vi "WPI_AnalogChannelVoltageToValue.vi"(6 "Relative":bool, 8 "error in (no error)":errorcluster, 9 "Averaged":bool, 10 "Voltage":dbl, 11 "AIDeviceRef":T1={"DevStatus"={"status"=FALSE, "code"=0, "source"=""}, "Analog Channel"=enum."AI 1"}) -> (0 "error out":errorcluster, 2 "Value":i32, 3 "AIDeviceRef":T1={"DevStatus"={"status"=FALSE, "code"=0, "source"=""}, "Analog Channel"=enum."AI 1"})   [LabVIEW 2017]
uses:
  <vilib>/Rock Robotics/WPI/AnalogChannel/WPI_AnalogChannelDevRef.ctl
  <vilib>/Rock Robotics/SystemInterfaces/AI/FPGA_AIChannel.ctl
  <vilib>/Rock Robotics/SystemInterfaces/System/FPGA_SystemGet.vi
  <vilib>/Rock Robotics/SystemInterfaces/AI/FPGA_AIOversampleBits.vi
  <vilib>/Rock Robotics/SystemInterfaces/AI/FPGA_AIERRInvalidAnalogChannel.vi
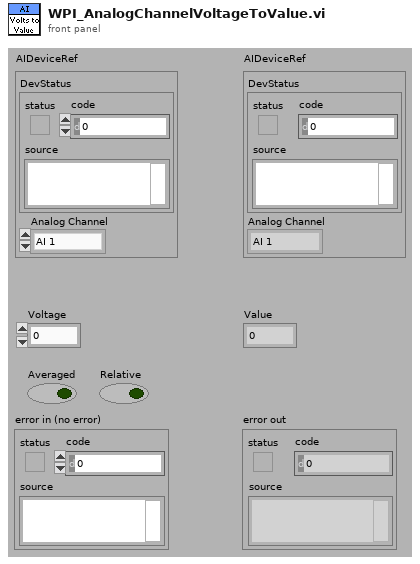
[diagram p1: front panel]
types:
  T1 = typedef "WPI_AnalogChannelDevRef.ctl" = cluster{"DevStatus":errorcluster, "Analog Channel":T2}
  T2 = typedef "FPGA_AIChannel.ctl" = enum8{"AI 0", "AI 1", "AI 2", "AI 3", "AI MXP 0", "AI MXP 1", "AI MXP 2", "AI MXP 3", "Invalid"}
  T3 = typedef "FPGA_AIDevRef.ctl" = cluster{"DevStatus":errorcluster}
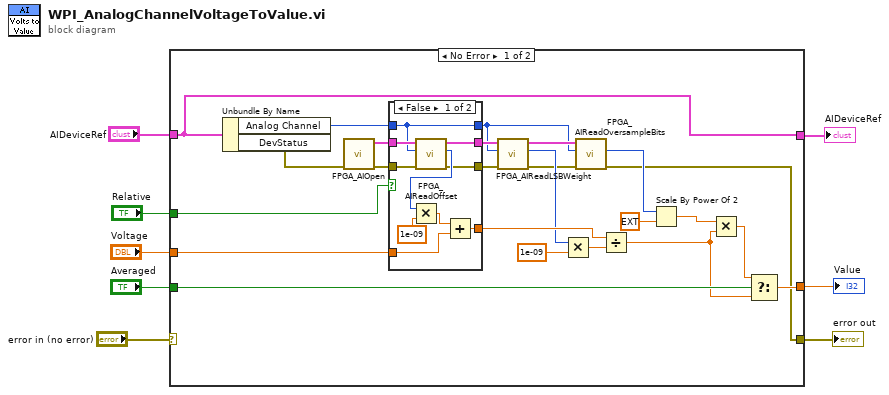
[diagram p0: block diagram]
diagram:
  n1 = case shown="No Error" "error in (no error)" {
    selector: "error in (no error)" -> [_ w47]
    tunnel: "Averaged" -> [w32 _]
    tunnel: [w31 _] -> w7
    tunnel: "Voltage" -> [w30 _]
    tunnel: "AIDeviceRef" -> [w17 w48]
    tunnel: [w17 w48] -> w3
    tunnel: [w16 w47] -> w2
    tunnel: "Relative" -> [w13 _]
    frame No Error {
      n2 = Unbundle By Name(w17) -> ("Analog Channel"=w29:T2, "DevStatus"=w12:errorcluster)
      n3 = call <vilib>:"FPGA_AIOpen.vi"("error in (no error)"=w12) -> ("error out"=w11:errorcluster, "AI Reference out"=w18:T3)  [unwired: 2 in, 7 out]
      n4 = case shown="False" w13 {
        tunnel: w30 -> [w42 w44]
        tunnel: w29 -> [w36 w45]
        tunnel: [w41 w44] -> w21
        tunnel: [w38 w46] -> w19
        tunnel: w18 -> [w37 w46]
        tunnel: [w36 w45] -> w15
        tunnel: w11 -> [w34 w43]
        tunnel: [w33 w43] -> w10
        frame False {
          n5 = call <vilib>:"FPGA_AIReadOffset.vi"("error in (no error)"=w34, "Channel"=w36, "AI Reference"=w37) -> ("error out"=w33:errorcluster, "Offset"=w39:i32, "AI Reference"=w38:T3)  [unwired: 6 out]
          n6 = Multiply(x=w39, y=1e-09) -> (x*y=w40:dbl)
          n7 = Add(x=w40, y=w42) -> (x+y=w41:dbl)
        }
        frame True {
        }
      }
      n8 = call <vilib>:"FPGA_AIReadLSBWeight.vi"("error in (no error)"=w10, "Channel"=w15, "AI Reference"=w19) -> ("error out"=w9:errorcluster, "LSBWeight"=w20:u32, "AI Reference"=w23:T3)  [unwired: 6 out]
      n9 = Multiply(x=w20, y=1e-09) -> (x*y=w22:dbl)
      n10 = call <vilib>:"FPGA_AIReadOversampleBits.vi"("error in (no error)"=w9, "Channel"=w15, "AI Reference in"=w23) -> ("error out"=w16:errorcluster, "OversampleBits"=w27:u8)  [unwired: 1 in, 6 out]
      n11 = Divide(x=w21, y=w22) -> (x/y=w25:dbl)
      n12 = Scale By Power Of 2(n=w27, x=ext 1.0) -> (x*2^n=w26:ext)
      n13 = Multiply(x=w26, y=w25) -> (x*y=w24:ext)
      n14 = Select(t=w24, s=w32, f=w25) -> (s? t:f=w31:ext)
    }
    frame Error {
    }
  }
  "Value" <- w7
  "error out" <- w2
  "AIDeviceRef" <- w3
